vi "FindCoordTemplate.vi"(7 "FindAction":enum16{"FromTemp", "FromData"}(ring), 8 "error in (no error)":errorcluster, 10 "Project":string, 11 "Root In":path) -> (0 "error out":errorcluster, 1 "CoordTemplatePaths":path[](array[path]), 3 "Root Out":path)   [LabVIEW 2019]
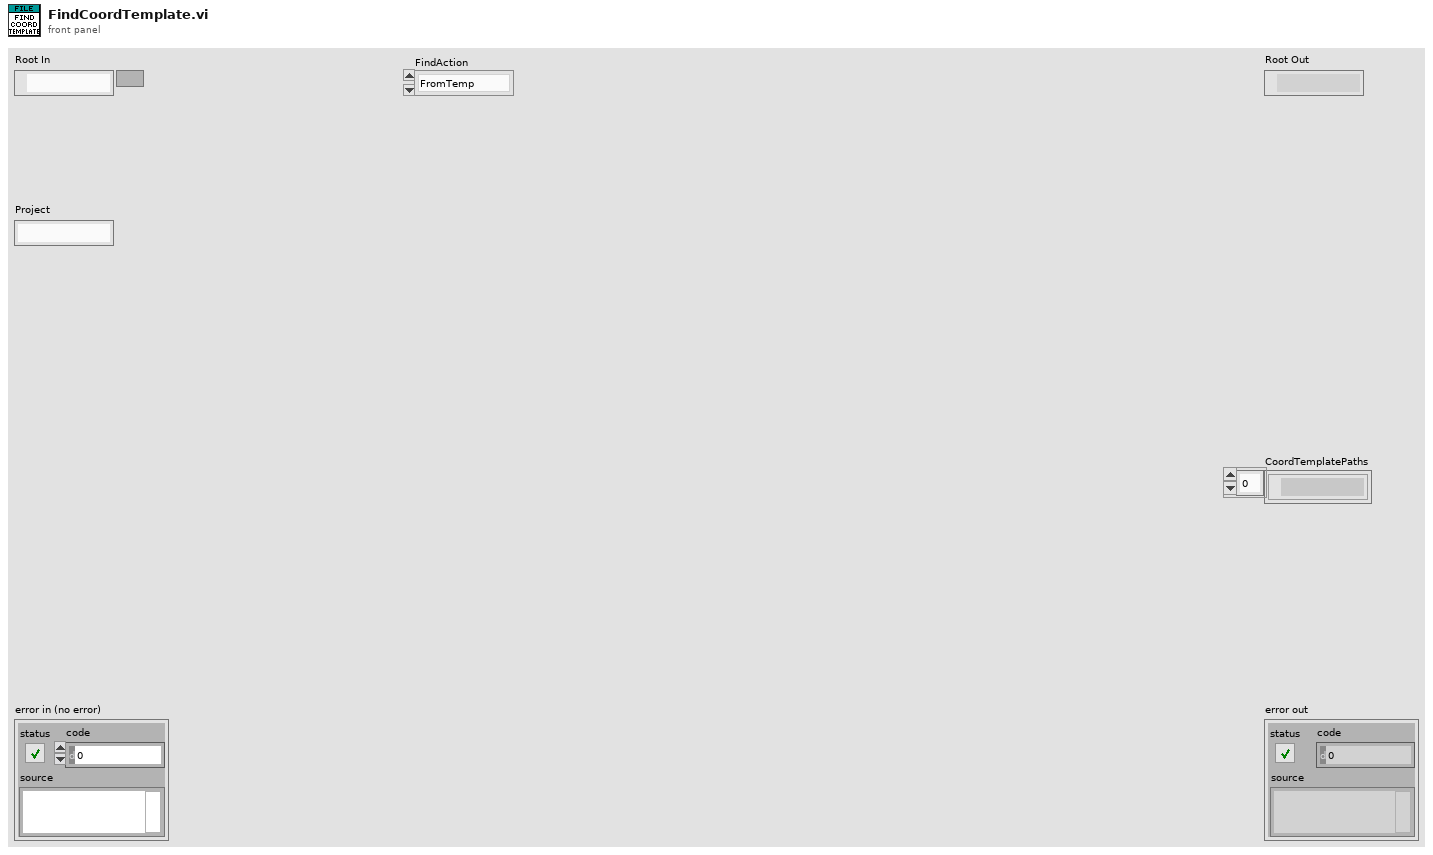
[diagram p1: front panel]
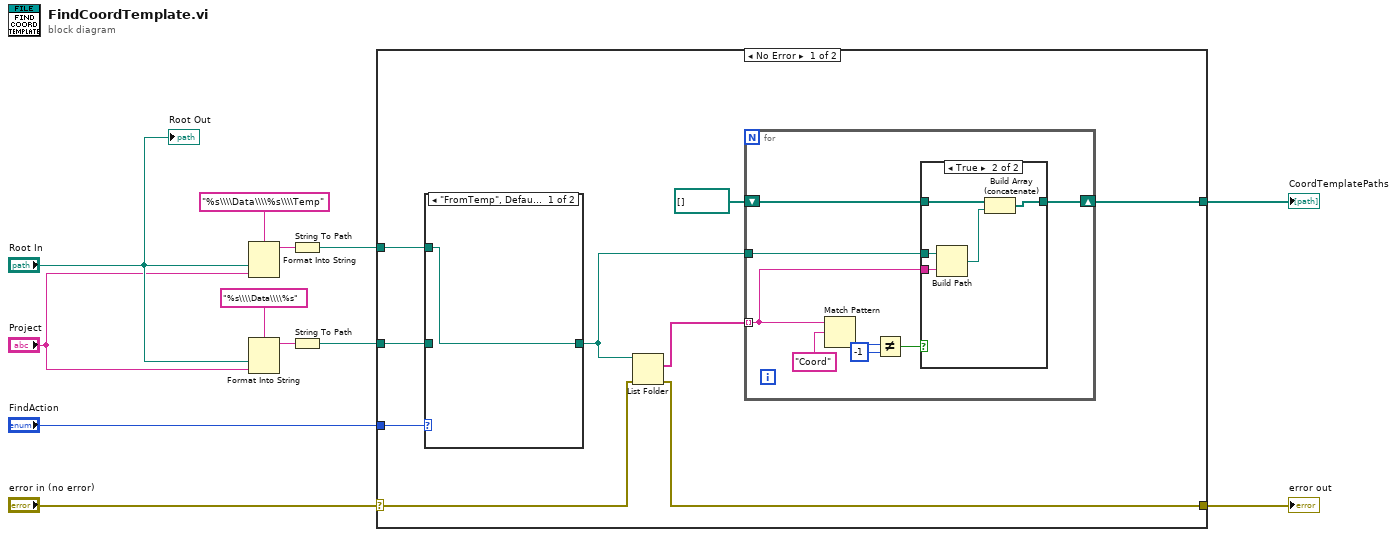
[diagram p0: block diagram]
diagram:
  n1 = Format Into String(format string="%s\\\\Data\\\\%s\\\\Temp", "Root In", "Project") -> (resulting string=w9:string)  [unwired: 2 in, 1 out]
  n2 = Format Into String(format string="%s\\\\Data\\\\%s", "Root In", "Project") -> (resulting string=w7:string)  [unwired: 2 in, 1 out]
  n3 = String To Path(string=w9) -> (path=w5:path)
  n4 = String To Path(string=w7) -> (path=w2:path)
  n5 = case shown="No Error" "error in (no error)" {
    selector: "error in (no error)" -> [w21 w38]
    tunnel: w5 -> [w15 _]
    tunnel: [w20 w38] -> w11
    tunnel: [w17 _] -> w10
    tunnel: w2 -> [w14 _]
    tunnel: "FindAction" -> [w16 _]
    frame No Error {
      n6 = case shown="\"FromTemp\", Default" w16 {
        tunnel: w15 -> [w22 _]
        tunnel: w14 -> [_ w23]
        tunnel: [w22 w23] -> w13
        frame "FromTemp", Default {
        }
        frame "FromData" {
        }
      }
      n7 = List Folder(path=w13, error in=w21) -> (filenames=w18:string[], error out=w20:errorcluster)  [unwired: 2 in, 2 out]
      n8 = for {
        tunnel: w18 -> [w26] mode=indexing
        tunnel: w13 -> [w24]
        shift-right: [w25] -> w17
        shift-left: path[] [] -> [w27]
        n9 = Match Pattern(string=w26, regular expression="Coord") -> (offset past match=w30:i32)  [unwired: 1 in, 3 out]
        n10 = Not Equal?(x=w30, y=-1) -> (x != y?=w28:bool)
        n11 = case shown="True" w28 {
          tunnel: w27 -> [w32 w37]
          tunnel: w26 -> [_ w34]
          tunnel: [w32 w36] -> w25
          tunnel: w24 -> [_ w35]
          frame False {
          }
          frame True {
            n12 = Build Path(base path=w35, name or relative path=w34) -> (appended path=w33:path)
            n13 = Build Array (concatenate)(w37, w33) -> (w36:path[])
          }
        }
      }
    }
    frame Error {
    }
  }
  "error out" <- w11
  "CoordTemplatePaths" <- w10
  "Root Out" <- "Root In"
